vi "UseDefaultIfUnwired.vi"() -> ()   [LabVIEW 2019]
panel:
  in  "Numeric":u8
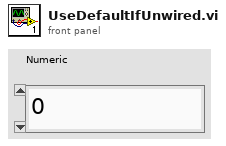
[diagram p1: front panel]
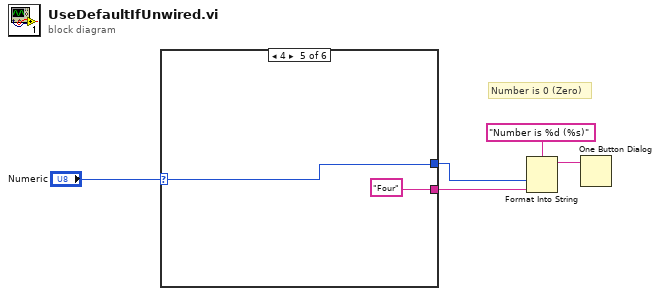
[diagram p0: block diagram]
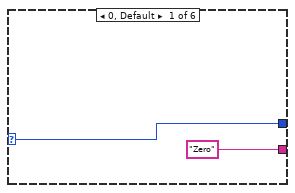
[diagram p2: hidden frame]
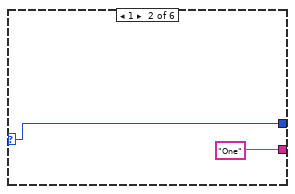
[diagram p3: hidden frame]
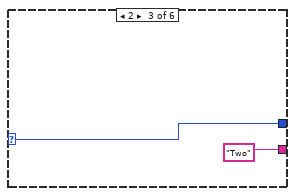
[diagram p4: hidden frame]
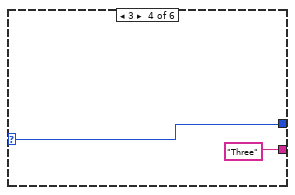
[diagram p5: hidden frame]
diagram:
  # "Number is 0 (Zero)"
  n1 = case shown="4" "Numeric" {
    selector: "Numeric" -> [w6 w8 w10 w12 w14 _]
    tunnel: ["Zero" "One" "Two" "Three" "Four" _] -> w2
    tunnel: [w6 w8 w10 w12 w14 _] -> w1
    frame 0, Default {
    }
    frame 1 {
    }
    frame 2 {
    }
    frame 3 {
    }
    frame 4 {
    }
    frame 5 {
    }
  }
  n2 = Format Into String(format string="Number is %d (%s)", w1, w2) -> (resulting string=w4:string)  [unwired: 2 in, 1 out]
  n3 = One Button Dialog(message=w4) -> ()  [unwired: 1 in, 1 out]
